vi "GetGobjectRefnums__slk_mt.vi"(8 "error in (no error)":errorcluster, 10 "from (Selected)":enum16{"All", "Selected"}(ring)=enum."Selected", 11 "vi refnum in":refnum<vi>) -> (0 "error out":errorcluster, 3 "generic objects refnums out":refnum<vi>[](array[refnum]))   [LabVIEW 2020, in "Lazyboots Menu Tool.lvlib"]
doc: "Gets generic objects refnums"
uses:
  Library/Lazyboots Menu Tool.lvlib
  TypeDef/TypeDef_GetGObjectRefnumsState__slk_mt.ctl
panel:
  # "GetGobjectRefnums__slk_mt.vi\nGets generic objects refnums\n\nNOTICE -- YOU MUST LEAVE THIS NOTICE IN PLACE.\n\nCopyright (c) 2011, LIANG LIU Shawn.Liu.cn@gmail.com\nAll rights reserved.\n\nRedistribution and use in source and binary forms, with or without modification, are permitted provided that the following conditions are met:\n-Redistributions of source code must retain the above copyright notice, this list of conditions and the following disclaimer.\n-Redistributions in binary form must reproduce the above copyright notice, this list of conditions and the following disclaimer in the documentation and/or other materials provided with the distribution.\n-Neither the name of the eLp nor the names of its contributors may be used to endorse or promote products derived from this software without specific prior written permission.\n\nTHIS SOFTWARE IS PROVIDED BY THE COPYRIGHT HOLDERS AND CONTRIBUTORS \"AS IS\" AND ANY EXPRESS OR IMPLIED WARRANTIES, INCLUDING, BUT NOT LIMITED TO, THE IMPLIED WARRANTIES OF MERCHANTABILITY AND FITNESS FOR A PARTICULAR PURPOSE ARE DISCLAIMED. IN NO EVENT SHALL THE COPYRIGHT HOLDER OR CONTRIBUTORS BE LIABLE FOR ANY DIRECT, INDIRECT, INCIDENTAL, SPECIAL, EXEMPLARY, OR CONSEQUENTIAL DAMAGES (INCLUDING, BUT NOT LIMITED TO, PROCUREMENT OF SUBSTITUTE GOODS OR SERVICES; LOSS OF USE, DATA, OR PROFITS; OR BUSINESS INTERRUPTION) HOWEVER CAUSED AND ON ANY THEORY OF LIABILITY, WHETHER IN CONTRACT, STRICT LIABILITY, OR TORT (INCLUDING NEGLIGENCE OR OTHERWISE) ARISING IN ANY WAY OUT OF THE USE OF THIS SOFTWARE, EVEN IF ADVISED OF THE POSSIBILITY OF SUCH DAMAGE."
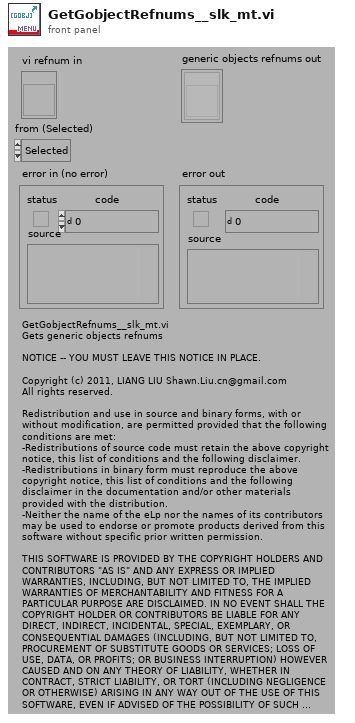
[diagram p1: front panel]
types:
  T1 = typedef "Lazyboots Menu Tool.lvlib/TypeDef_GetGObjectRefnumsState__slk_mt.ctl" = enum16{"From?", "Get FP Selected", "Get BD Selected", "Concatenate FP and BD", "Get All", "End"}
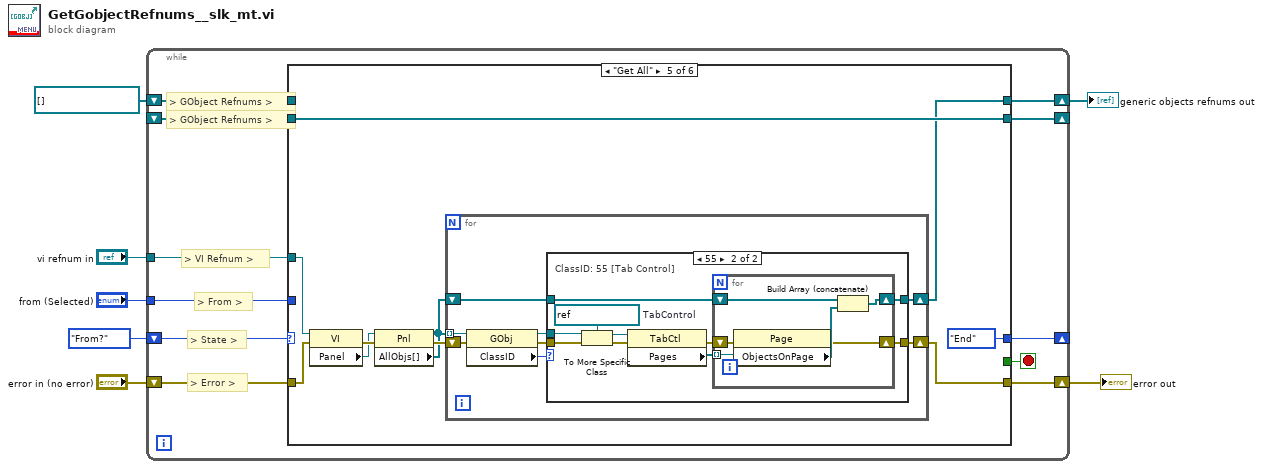
[diagram p0: block diagram]
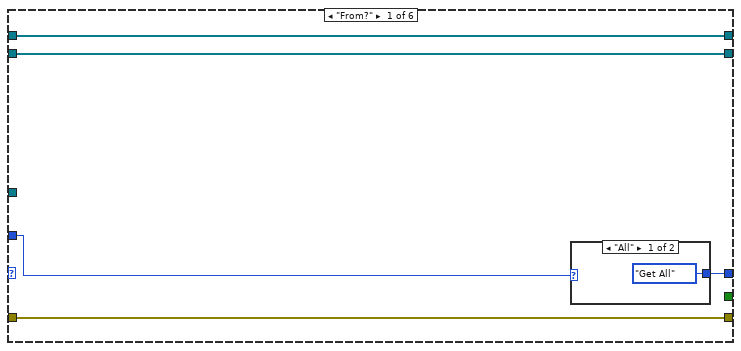
[diagram p2: hidden frame]
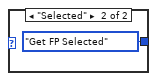
[diagram p3: hidden frame]
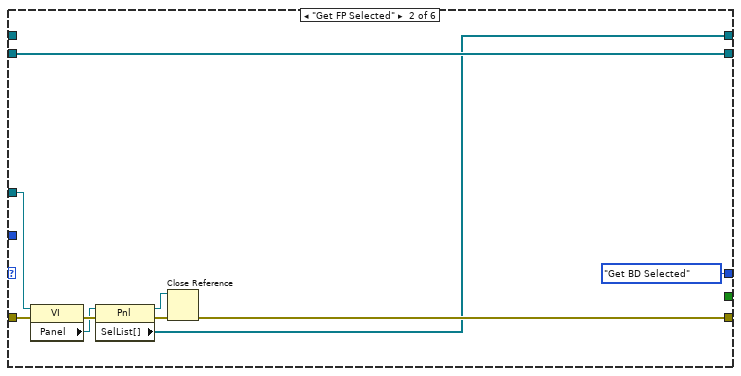
[diagram p4: hidden frame]
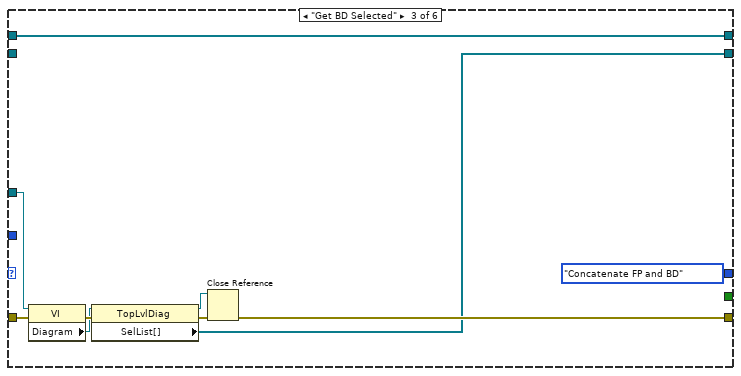
[diagram p5: hidden frame]
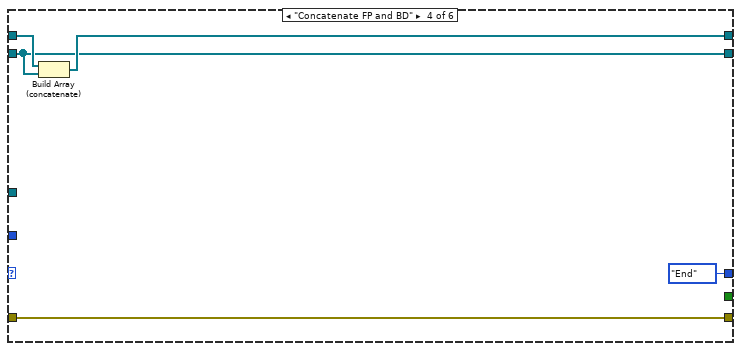
[diagram p6: hidden frame]
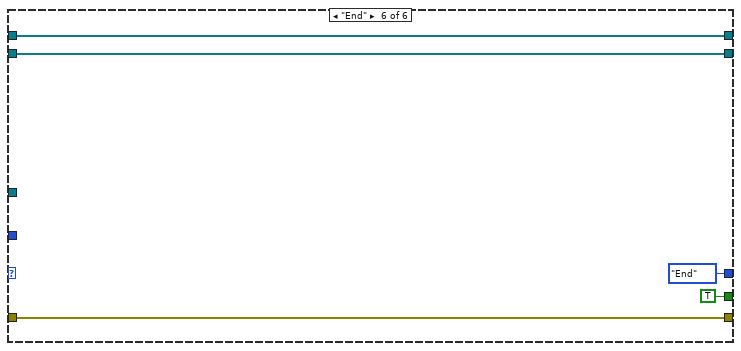
[diagram p8: hidden frame]
diagram:
  n1 = while {
    shift-right: [w16] -> w6
    shift-left: "error in (no error)" -> [w17]
    shift-right: [w9] -> _
    shift-left: TypeDef_GetGObjectRefnumsState__slk_mt."From?" ("State") -> [w18]
    shift-right: [w13] -> _
    shift-left: _ -> [w14]
    tunnel: "from (Selected)" -> [w12]
    shift-right: [w11] -> w2
    shift-left: refnum<vi>[] [] ("SelList[]") -> [w15]
    tunnel: "vi refnum in" -> [w10]
    stop <- w8 stop-if-true
    # "> From >"
    # "> VI Refnum >"
    # "> GObject Refnums >"
    # "> GObject Refnums >"
    # "> Error >"
    # "> State >"
    n2 = case shown="\"Get All\"" w18 {
      tunnel: w17 -> [w23 w35 w45 w48 w60 w88]
      tunnel: [w23 w29 w40 w48 w53 w88] -> w16
      tunnel: w15 -> [w22 _ w37 w49 _ w91]
      tunnel: [w22 w26 w37 w47 w51 w91] -> w11
      tunnel: w14 -> [w21 w34 _ w46 w59 w90]
      tunnel: [w21 w34 w36 w46 w59 w90] -> w13
      tunnel: w12 -> [w20 _ _ _ _ _]
      tunnel: w10 -> [_ w32 w43 _ w57 _]
      tunnel: [w19 TypeDef_GetGObjectRefnumsState__slk_mt."Get BD Selected" ("State") TypeDef_GetGObjectRefnumsState__slk_mt."Concatenate FP and BD" ("State") TypeDef_GetGObjectRefnumsState__slk_mt."End" ("State") TypeDef_GetGObjectRefnumsState__slk_mt."End" ("State") TypeDef_GetGObjectRefnumsState__slk_mt."End" ("State")] -> w9
      tunnel: [_ _ _ _ _ TRUE] -> w8
      frame "From?" {
        n3 = case shown="\"All\"" w20 {
          tunnel: [TypeDef_GetGObjectRefnumsState__slk_mt."Get All" ("State") TypeDef_GetGObjectRefnumsState__slk_mt."Get FP Selected" ("State")] -> w19
          frame "All" {
          }
          frame "Selected" {
          }
        }
      }
      frame "Get FP Selected" {
        n4 = property class="VI"(reference=w32, error in=w35) -> (error out=w33:errorcluster, "Panel"=w30:refnum<vi>)  [unwired: 1 out]
        n5 = property class="Pnl"(reference=w30, error in=w33) -> (reference out=w28:refnum<vi>, error out=w31:errorcluster, "SelList[]"=w26:refnum<vi>[])
        n6 = Close Reference(reference=w28, error in (no error)=w31) -> (error out=w29:errorcluster)
      }
      frame "Get BD Selected" {
        n7 = property class="VI"(reference=w43, error in=w45) -> (error out=w44:errorcluster, "Diagram"=w41:refnum<vi>)  [unwired: 1 out]
        n8 = property class="TopLvlDiag"(reference=w41, error in=w44) -> (reference out=w39:refnum<vi>, error out=w42:errorcluster, "SelList[]"=w36:refnum<vi>[])
        n9 = Close Reference(reference=w39, error in (no error)=w42) -> (error out=w40:errorcluster)
      }
      frame "Concatenate FP and BD" {
        n10 = Build Array (concatenate)(w49, w46) -> (w47:refnum<vi>[])
      }
      frame "Get All" {
        n11 = property class="VI"(reference=w57, error in=w60) -> (error out=w58:errorcluster, "Panel"=w56:refnum<vi>)  [unwired: 1 out]
        n12 = property class="Pnl"(reference=w56, error in=w58) -> (error out=w54:errorcluster, "AllObjs[]"=w52:refnum<vi>[])  [unwired: 1 out]
        n13 = for {
          shift-right: [w62] -> w51
          shift-left: w52 -> [w64]
          shift-right: [w63] -> w53
          shift-left: w54 -> [w68]
          tunnel: w52 -> [w61] mode=indexing
          n14 = property class="GObj"(reference=w61, error in=w68) -> (reference out=w66:refnum<vi>, error out=w65:errorcluster, "ClassID"=w67:u32)
          n15 = case shown="55" w67 {
            tunnel: w66 -> [_ w78]
            tunnel: w65 -> [w70 w80]
            tunnel: w64 -> [w69 w73]
            tunnel: [w70 w72] -> w63
            tunnel: [w69 w71] -> w62
            frame Default {
            }
            frame 55 {
              w76 = refnum<vi> refnum  # TabControl
              # "ClassID: 55 [Tab Control]"
              n16 = To More Specific Class(target class=w76, reference=w78, error in=w80) -> (specific class reference=w77:refnum<vi>, error out=w79:errorcluster)
              n17 = property class="TabCtl"(reference=w77, error in=w79) -> (error out=w74:errorcluster, "Pages"=w75:refnum<vi>[])  [unwired: 1 out]
              n18 = for {
                tunnel: w75 -> [w85] mode=indexing
                shift-right: [w83] -> w71
                shift-left: w73 -> [w84]
                shift-right: [w81] -> w72
                shift-left: w74 -> [w86]
                n19 = property class="Page"(reference=w85, error in=w86) -> (error out=w81:errorcluster, "ObjectsOnPage"=w82:refnum<vi>[])  [unwired: 1 out]
                n20 = Build Array (concatenate)(w84, w82) -> (w83:refnum<vi>[])
              }
            }
          }
        }
      }
      frame "End" {
      }
    }
  }
  "error out" <- w6
  "generic objects refnums out" <- w2
